vi "Read Configuration.vi"(8 "error in (no error)":errorcluster, 11 "Report Generator In":refnum<class "Report Generator.lvclass">) -> (0 "error out":errorcluster, 3 "Report Generator Out":refnum<class "Report Generator.lvclass">)   [LabVIEW 2020, in "Report Generator.lvclass"]
doc: "Method that read any necessay configurations from config file or potentially configure hard coded values. s"
uses:
  Report Generator.lvclass
  Report Generator.lvclass/Report Generator.ctl
  Application Framework/Support/Configuration File/Configuration File.lvlib
  Report Classes/Test Report/Test Report.lvclass
  Report Classes/XML Report/XML Report.lvclass
  C:/Users/anton/Documents/GitHub/LUnit/source/Application Framework/Process Classes/Process/Process.lvclass
  C:/Users/anton/Documents/GitHub/LUnit/source/Framework/Report Generator/Report Generator.lvclass
  C:/Users/anton/Documents/GitHub/LUnit/source/Framework/Report Classes/Test Report/Test Report.lvclass
  C:/Users/anton/Documents/GitHub/LUnit/source/Framework/Report Classes/XML Report/XML Report.lvclass
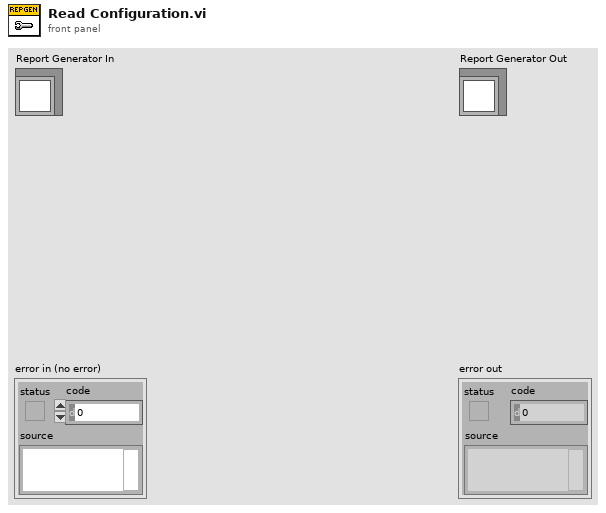
[diagram p1: front panel]
types:
  T1 = typedef "NI_LVConfig.lvlib/Config Data RefNum.ctl" = refnum<k1>
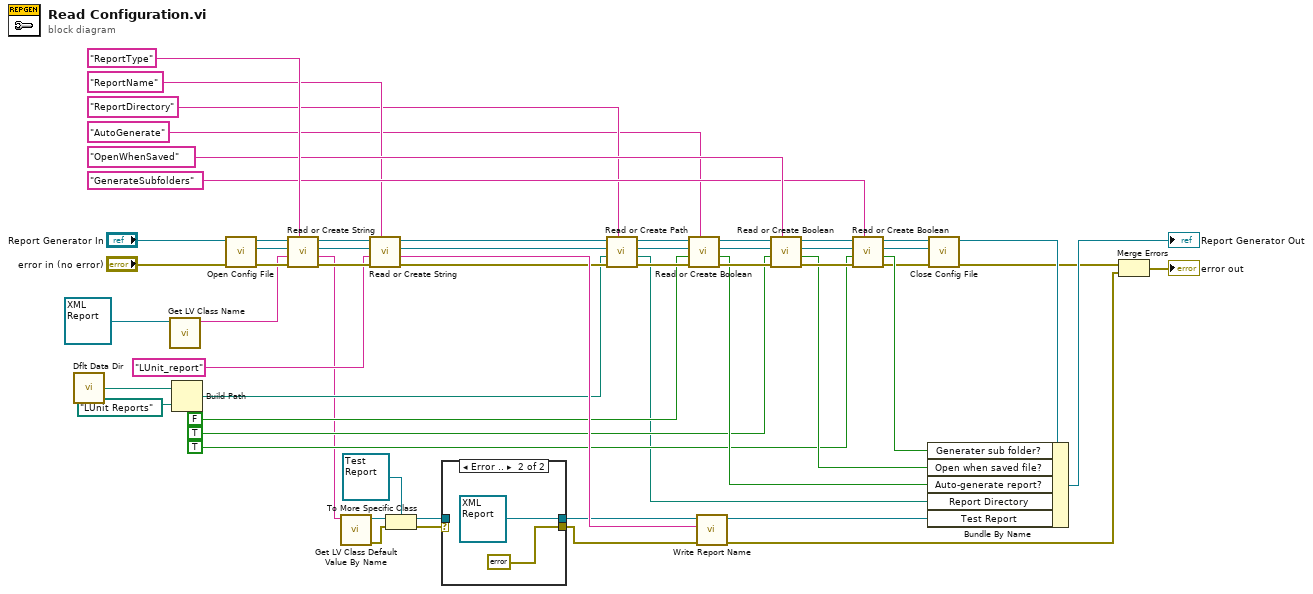
[diagram p0: block diagram]
diagram:
  n1 = call <vilib>:"Dflt Data Dir.vi"() -> ("App:Default Data Directory"=w37:path)
  n2 = call <vilib>:"Get LV Class Name.vi"("object"=refnum<class "XML Report.lvclass"> refnum ("XML Report.lvclass")) -> ("class name"=w6:string)  [unwired: 9 in, 1 out]
  n3 = Build Path(base path=w37, name or relative path=path "LUnit Reports") -> (appended path=w35:path)
  n4 = call "Open Config File.vi"("error in (no error)"="error in (no error)", "Process in"="Report Generator In") -> ("error out"=w29:errorcluster, "refnum out"=w25:T1, "Process out"=w30:refnum<class "Report Generator.lvclass">)  [unwired: 6 in, 1 out]
  n5 = call "Read or Create String.vi"("key"="ReportType", "error in (no error)"=w29, "default value"=w6, "refnum"=w25, "Process in"=w30) -> ("error out"=w43:errorcluster, "value"=w12:string, "refnum out"=w24:T1, "Process out"=w44:refnum<class "Report Generator.lvclass">)  [unwired: 3 in]
  n6 = call <vilib>:"Get LV Class Default Value By Name.vi"("class name"=w12) -> ("error out"=w9:errorcluster, "object"=w11:refnum<class>)  [unwired: 9 in]
  n7 = call "Read or Create String.vi"("key"="ReportName", "error in (no error)"=w43, "default value"="LUnit_report", "refnum"=w24, "Process in"=w44) -> ("error out"=w41:errorcluster, "value"=w48:string, "refnum out"=w23:T1, "Process out"=w42:refnum<class "Report Generator.lvclass">)  [unwired: 3 in]
  n8 = To More Specific Class(target class=refnum<class "Test Report.lvclass"> refnum ("Test Report.lvclass"), reference=w11, error in=w9) -> (specific class reference=w2:refnum<class "Test Report.lvclass">, error out=w5:errorcluster)
  n9 = case shown="Error .." w5 {
    selector: w5 -> [w59 _]
    tunnel: [w59 errorcluster {"status"=FALSE, "code"=0, "source"=""} ("error IO")] -> w4
    tunnel: [w58 refnum<class "XML Report.lvclass"> refnum ("XML Report.lvclass")] -> w3
    tunnel: w2 -> [w58 _]
    frame No Error {
    }
    frame Error {
    }
  }
  n10 = call "Read or Create Path.vi"("key"="ReportDirectory", "error in (no error)"=w41, "default value"=w35, "refnum"=w23, "Process in"=w42) -> ("error out"=w39:errorcluster, "value"=w31:path, "refnum out"=w22:T1, "Process out"=w40:refnum<class "Report Generator.lvclass">)  [unwired: 3 in]
  n11 = call "Read or Create Boolean.vi"("key"="AutoGenerate", "error in (no error)"=w39, "default value"=FALSE, "refnum"=w22, "Process in"=w40) -> ("error out"=w54:errorcluster, "value"=w45:bool, "refnum out"=w21:T1, "Process out"=w53:refnum<class "Report Generator.lvclass">)  [unwired: 3 in]
  n12 = call "Write Report Name.vi"("error in (no error)"=w4, "Report Name"=w48, "Report In"=w3) -> ("error out"=w7:errorcluster, "Report Out"=w49:refnum<class "Test Report.lvclass">)  [unwired: 7 in]
  n13 = call "Read or Create Boolean.vi"("key"="OpenWhenSaved", "error in (no error)"=w54, "default value"=TRUE, "refnum"=w21, "Process in"=w53) -> ("error out"=w50:errorcluster, "value"=w46:bool, "refnum out"=w20:T1, "Process out"=w52:refnum<class "Report Generator.lvclass">)  [unwired: 3 in]
  n14 = call "Read or Create Boolean.vi"("key"="GenerateSubfolders", "error in (no error)"=w50, "default value"=TRUE, "refnum"=w20, "Process in"=w52) -> ("error out"=w27:errorcluster, "value"=w47:bool, "refnum out"=w19:T1, "Process out"=w51:refnum<class "Report Generator.lvclass">)  [unwired: 3 in]
  n15 = call "Close Config File.vi"("error in (no error)"=w27, "refnum"=w19, "Process in"=w51) -> ("error out"=w26:errorcluster, "Process out"=w28:refnum<class "Report Generator.lvclass">)  [unwired: 6 in, 1 out]
  n16 = Bundle By Name(cluster=w28, "Generater sub folder?"=w47, "Open when saved file?"=w46, "Auto-generate report?"=w45, "Report Directory"=w31, "Test Report"=w49) -> (→"Report Generator Out":refnum<class "Report Generator.lvclass">)
  n17 = Merge Errors(w26, w7) -> (→"error out":errorcluster)
